vi "Check_and_Update_Crop_CFG.vi"(9 "Y resolution":i32, 10 "X resolution":i32, 11 "Crop_CFG_In":T1) -> (2 "Valid?":bool, 3 "Crop_CFG_Out":T1)   [LabVIEW 2020]
uses:
  <vilib>/Ngene/DeepLTK Anomaly Detection Addon/Toolkit/API/Controls/Crop_CFG.ctl
  <vilib>/Ngene/DeepLTK Anomaly Detection Addon/Toolkit/DeepLTK_Anomaly_Detection_Addon.lvlib
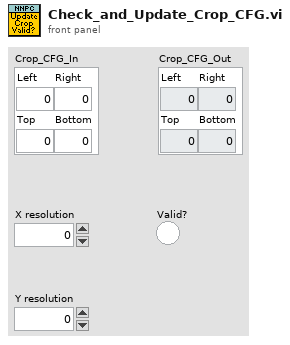
[diagram p1: front panel]
types:
  T1 = typedef "DeepLTK_Anomaly_Detection_Addon.lvlib/Crop_CFG.ctl" = cluster{"Left":sgl, "Top":sgl, "Right":sgl, "Bottom":sgl}
  T2 = cluster{"Left":bool, "Top":bool, "Right":bool, "Bottom":bool}
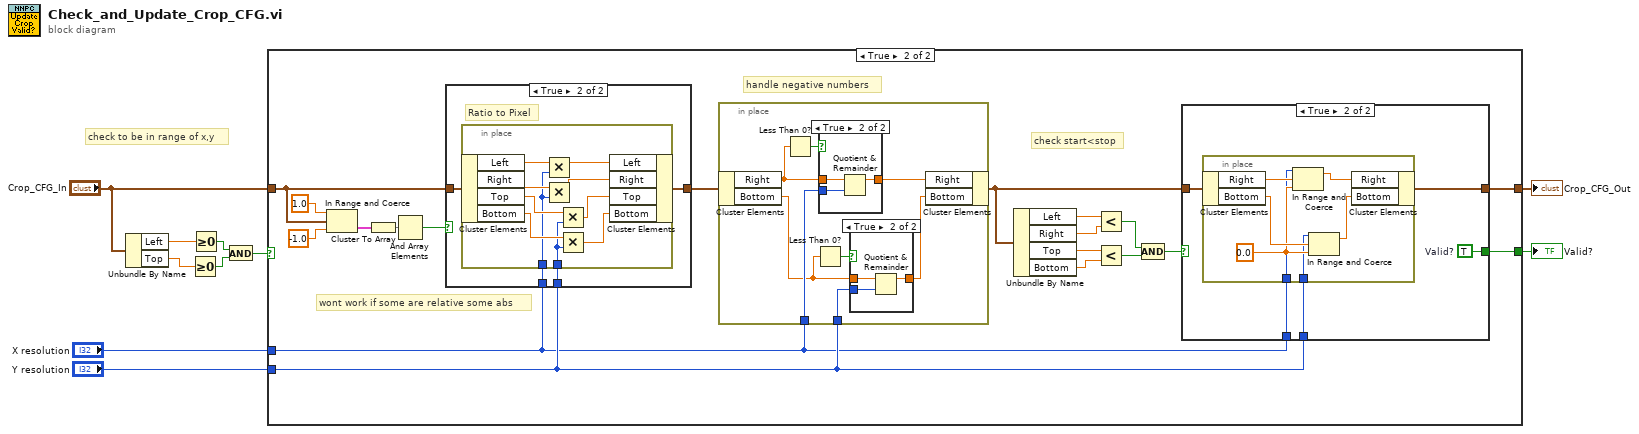
[diagram p0: block diagram]
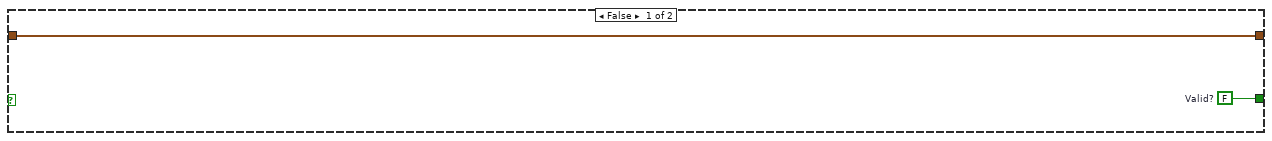
[diagram p2: hidden frame]
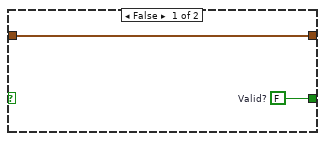
[diagram p3: hidden frame]
diagram:
  # "check to be in range of x,y"
  n1 = Unbundle By Name("Crop_CFG_In") -> ("Left"=w7:sgl, "Top"=w8:sgl)
  n2 = Greater Or Equal To 0?(x=w8) -> (x >= 0?=w10:bool)
  n3 = Greater Or Equal To 0?(x=w7) -> (x >= 0?=w9:bool)
  n4 = And(x=w9, y=w10) -> (x .and. y?=w6:bool)
  n5 = case shown="True" w6 {
    tunnel: "X resolution" -> [_ w14]
    tunnel: "Y resolution" -> [_ w15]
    tunnel: "Crop_CFG_In" -> [w12 w23]
    tunnel: [w12 w16] -> w2
    tunnel: [w11 w13] -> w1
    frame False {
      w11 = FALSE  # Valid?
    }
    frame True {
      # "check start<stop"
      # "handle negative numbers"
      # "wont work if some are relative some abs"
      n6 = In Range and Coerce(upper limit=sgl 1.0 ("x*y"), x=w23, lower limit=sgl -1.0 ("x*y")) -> (In Range?=w31:T2)  [unwired: 1 out]
      n7 = Cluster To Array(cluster=w31) -> (array=w30:bool[])
      n8 = And Array Elements(Boolean array=w30) -> (logical AND=w29:bool)
      n9 = case shown="True" w29 {
        tunnel: w23 -> [w62 w66]
        tunnel: w14 -> [_ w65]
        tunnel: w15 -> [_ w64]
        tunnel: [w62 w63] -> w26
        frame False {
        }
        frame True {
          # "Ratio to Pixel"
          n10 = in-place {
            in-place-border: w65 -> [w68]
            in-place-border: w64 -> [w67]
            n11 = in-place-cluster #1(w66) -> ("Left"=w76:sgl, "Right"=w75:sgl, "Top"=w74:sgl, "Bottom"=w73:sgl)
            n12 = Multiply(x=w76, y=w68) -> (x*y=w72:sgl)
            n13 = Multiply(x=w75, y=w68) -> (x*y=w71:sgl)
            n14 = Multiply(x=w74, y=w67) -> (x*y=w70:sgl)
            n15 = Multiply(x=w73, y=w67) -> (x*y=w69:sgl)
            n16 = in-place-cluster #1("Left"=w72, "Right"=w71, "Top"=w70, "Bottom"=w69) -> (w63:T1)
          }
        }
      }
      n17 = in-place {
        in-place-border: w14 -> [w52]
        in-place-border: w15 -> [w49]
        n18 = in-place-cluster #2(w26) -> ("Right"=w51:sgl, "Bottom"=w46:sgl)
        n19 = Less Than 0?(x=w51) -> (x < 0?=w50:bool)
        n20 = Less Than 0?(x=w46) -> (x < 0?=w47:bool)
        n21 = case shown="True" w50 {
          tunnel: w51 -> [w58 w61]
          tunnel: [w58 w60] -> w53
          tunnel: w52 -> [_ w59]
          frame False {
          }
          frame True {
            n22 = Quotient & Remainder(x=w61, y=w59) -> (x-y*floor(x/y)=w60:sgl)  [unwired: 1 out]
          }
        }
        n23 = case shown="True" w47 {
          tunnel: w46 -> [w54 w57]
          tunnel: [w54 w56] -> w48
          tunnel: w49 -> [_ w55]
          frame False {
          }
          frame True {
            n24 = Quotient & Remainder(x=w57, y=w55) -> (x-y*floor(x/y)=w56:sgl)  [unwired: 1 out]
          }
        }
        n25 = in-place-cluster #2("Right"=w53, "Bottom"=w48) -> (w17:T1)
      }
      n26 = Unbundle By Name(w17) -> ("Left"=w25:sgl, "Right"=w22:sgl, "Top"=w24:sgl, "Bottom"=w21:sgl)
      n27 = Less?(x=w25, y=w22) -> (x < y?=w20:bool)
      n28 = Less?(x=w24, y=w21) -> (x < y?=w19:bool)
      n29 = Compound Arithmetic op=AND(w20, w19) -> (w18:bool)
      n30 = case shown="True" w18 {
        tunnel: w17 -> [w33 w38]
        tunnel: [w33 w37] -> w16
        tunnel: w15 -> [_ w36]
        tunnel: w14 -> [_ w35]
        tunnel: [w32 w34] -> w13
        frame False {
          w32 = FALSE  # Valid?
        }
        frame True {
          w34 = TRUE  # Valid?
          n31 = in-place {
            in-place-border: w36 -> [w39]
            in-place-border: w35 -> [w40]
            w41 = sgl 0.0 ("lower limit")
            n32 = in-place-cluster #3(w38) -> ("Right"=w45:sgl, "Bottom"=w44:sgl)
            n33 = In Range and Coerce(upper limit=w40, x=w45, lower limit=w41) -> (coerced(x)=w43:sgl)  [unwired: 1 out]
            n34 = In Range and Coerce(upper limit=w39, x=w44, lower limit=w41) -> (coerced(x)=w42:sgl)  [unwired: 1 out]
            n35 = in-place-cluster #3("Right"=w43, "Bottom"=w42) -> (w37:T1)
          }
        }
      }
    }
  }
  "Crop_CFG_Out" <- w2
  "Valid?" <- w1
